vi "Main.vi"() -> ()   [LabVIEW 2017]
uses:
  <userlib>/_NEVSTOP/Communicable State Machine(CSM)/Communicable State Machine.lvlib
panel:
  out "Settings":string="DoA"
  out "error out":errorcluster
  out "DataBool":string="DoA"
  out "DataString":string="DoA"
  out "Settings.Bool":string="DoA"
  out "Settings.String":string="DoA"
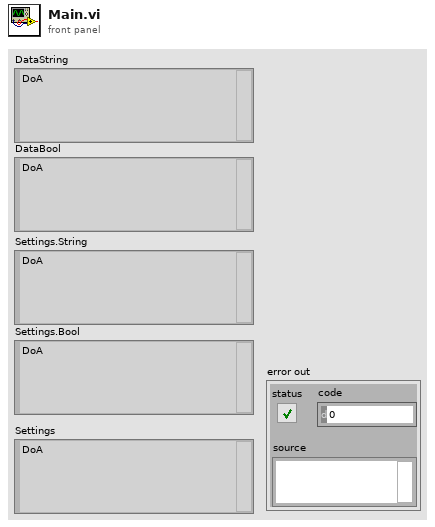
[diagram p1: front panel]
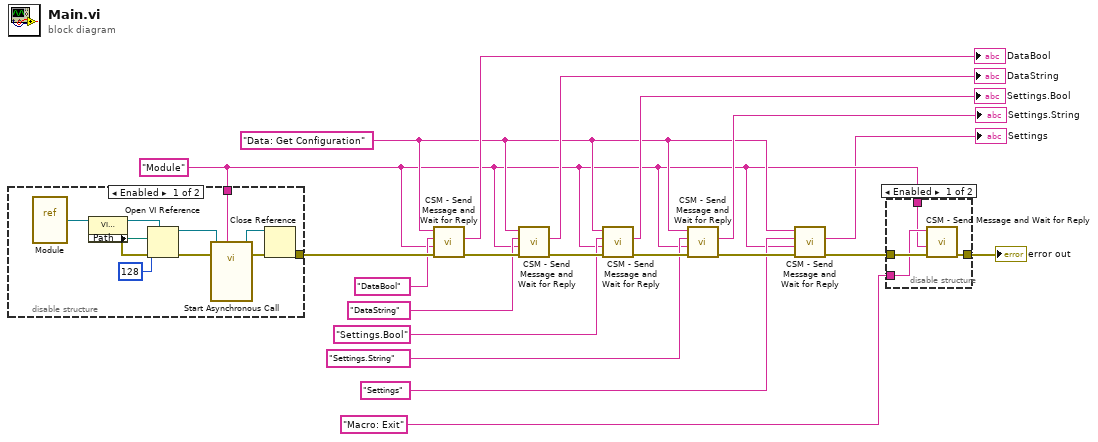
[diagram p0: block diagram]
diagram:
  w3 = "Data: Get Configuration" ("Name(\"\" to use uuid)")
  w2 = "Module" ("Name(\"\" to use uuid)")
  n1 = disable-structure shown="Enabled" {
    disable-tunnel: [w22 _] -> w20
    disable-tunnel: w2 -> [w21 _]
    frame Enabled {
      n2 = vi-ref "Module.vi"() -> (w25:refnum<vi>)
      n3 = property class="VI (strict)"(reference=w25) -> (reference out=w29:refnum<vi>, error out=w27:errorcluster, "Path"=w26:path)  [unwired: 1 in]
      n4 = Open VI Reference(type specifier VI Refnum (for type only)=w29, vi path=w26, options=128, error in (no error)=w27) -> (vi reference=w24:refnum<vi>, error out=w30:errorcluster)  [unwired: 2 in]
      n5 = call-by-ref "Start Asynchronous Call"(reference=w24, error in=w30, "Name(\"\" to use uuid)"=w21) -> (reference out=w23:refnum<vi>, error out=w28:errorcluster)  [unwired: 11 in]
      n6 = Close Reference(reference=w23, error in (no error)=w28) -> (error out=w22:errorcluster)
    }
    frame Disabled {
    }
  }
  n7 = call <userlib>:"CSM - Send Message and Wait for Reply.vi"("Error In (no error)"=w20, "Target Module"=w2, "Arguments (\"\")"="DataBool" ("Name(\"\" to use uuid)"), "State"=w3) -> ("error out"=w19:errorcluster, "Arguments"=→"DataBool":string)  [unwired: 6 in]
  n8 = call <userlib>:"CSM - Send Message and Wait for Reply.vi"("Error In (no error)"=w19, "Target Module"=w2, "Arguments (\"\")"="DataString" ("Name(\"\" to use uuid)"), "State"=w3) -> ("error out"=w17:errorcluster, "Arguments"=→"DataString":string)  [unwired: 6 in]
  n9 = call <userlib>:"CSM - Send Message and Wait for Reply.vi"("Error In (no error)"=w17, "Target Module"=w2, "Arguments (\"\")"="Settings.Bool" ("Name(\"\" to use uuid)"), "State"=w3) -> ("error out"=w18:errorcluster, "Arguments"=→"Settings.Bool":string)  [unwired: 6 in]
  n10 = call <userlib>:"CSM - Send Message and Wait for Reply.vi"("Error In (no error)"=w18, "Target Module"=w2, "Arguments (\"\")"="Settings.String" ("Name(\"\" to use uuid)"), "State"=w3) -> ("error out"=w6:errorcluster, "Arguments"=→"Settings.String":string)  [unwired: 6 in]
  n11 = call <userlib>:"CSM - Send Message and Wait for Reply.vi"("Error In (no error)"=w6, "Target Module"=w2, "Arguments (\"\")"="Settings" ("Name(\"\" to use uuid)"), "State"=w3) -> ("error out"=w5:errorcluster, "Arguments"=→"Settings":string)  [unwired: 6 in]
  n12 = disable-structure shown="Enabled" {
    disable-tunnel: w5 -> [w35 w36]
    disable-tunnel: [w34 w36] -> w8
    disable-tunnel: "Macro: Exit" ("Name(\"\" to use uuid)") -> [w33 _]
    disable-tunnel: w2 -> [w32 _]
    frame Enabled {
      n13 = call <userlib>:"CSM - Send Message and Wait for Reply.vi"("Error In (no error)"=w35, "Target Module"=w32, "State"=w33) -> ("error out"=w34:errorcluster)  [unwired: 7 in, 1 out]
    }
    frame Disabled {
    }
  }
  "error out" <- w8
